vi "Clock Deriver-3.vi"(10 "reset":bool, 11 "Divisor":u32=1 min=1) -> (2 "Clock Out":bool)   [LabVIEW 2013]
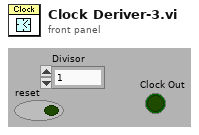
[diagram p1: front panel]
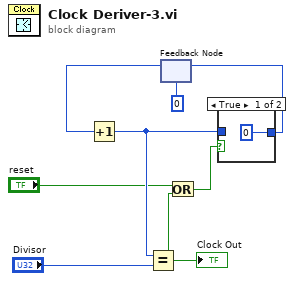
[diagram p0: block diagram]
diagram:
  n1 = feedback #1(u32 0) -> (w7:u32)
  n2 = Increment(x=w7) -> (x+1=w6:u32)
  n3 = Equal?(x=w6, y="Divisor") -> (x = y?=w5:bool)
  "Clock Out" <- w5
  n4 = Or(x="reset", y=w5) -> (x .or. y?=w2:bool)
  n5 = case shown="True" w2 {
    tunnel: [u32 0 w10] -> w3
    tunnel: w6 -> [_ w10]
    frame True {
    }
    frame False {
    }
  }
  n6 = feedback-in #1(w3) -> ()
